vi "GetServerVIName.vi"(1 "ROS":T1={"topic port"=0, "Node"="", "topic"="", "type"="", "node port"=0, "error "={"status"=FALSE, "code"=0, "source"=""}, "Direction"=enum."Node", "APIs"=[], "Update (ms)"=1, "write queue"=1}) -> (0 "vi name":string)   [LabVIEW 2012]
uses:
  _ROSControl.ctl
  _ROSDirection.ctl
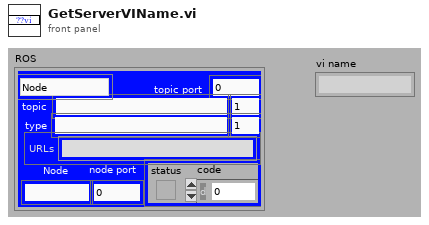
[diagram p1: front panel]
types:
  T1 = typedef "_ROSControl.ctl" = cluster{"topic port":u16, "Node":string, "topic":string, "type":string, "node port":u32, "error ":errorcluster, "Direction":T2, "APIs":string[], "Update (ms)":u16, "write queue":u16}
  T2 = typedef "_ROSDirection.ctl" = enum16{"Node", "Publisher", "Subscriber", "Service Client"}
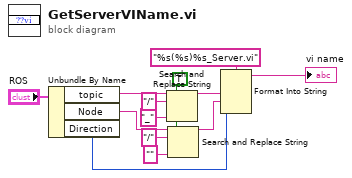
[diagram p0: block diagram]
diagram:
  w7 = TRUE ("replace all? (F)")
  n1 = Unbundle By Name("ROS") -> ("topic"=w11:string, "Node"=w12:string, "Direction"=w1:T2)
  n2 = Search and Replace String(replace all?=w7, input string=w11, search string="/" ("regular expression"), replace string="_" ("replace string (\"\")")) -> (result string=w5:string)  [unwired: 4 in, 3 out]
  n3 = Search and Replace String(replace all?=w7, input string=w12, search string="/" ("regular expression"), replace string="" ("replace string (\"\")")) -> (result string=w8:string)  [unwired: 4 in, 3 out]
  n4 = Format Into String(format string="%s(%s)%s_Server.vi", w5, w8, w1) -> (resulting string=→"vi name":string)  [unwired: 2 in, 1 out]
